vi "Checking_exe.vi"(8 "Task error in (no error)":errorcluster, 11 "Programes":string) -> (0 "Task error out":errorcluster, 3 "Game Running":bool=TRUE)   [LabVIEW 2014]
doc: "Check if an exe is running and optionally kill the process"
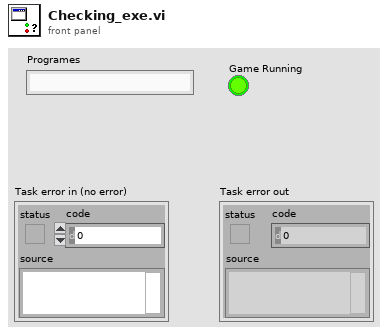
[diagram p1: front panel]
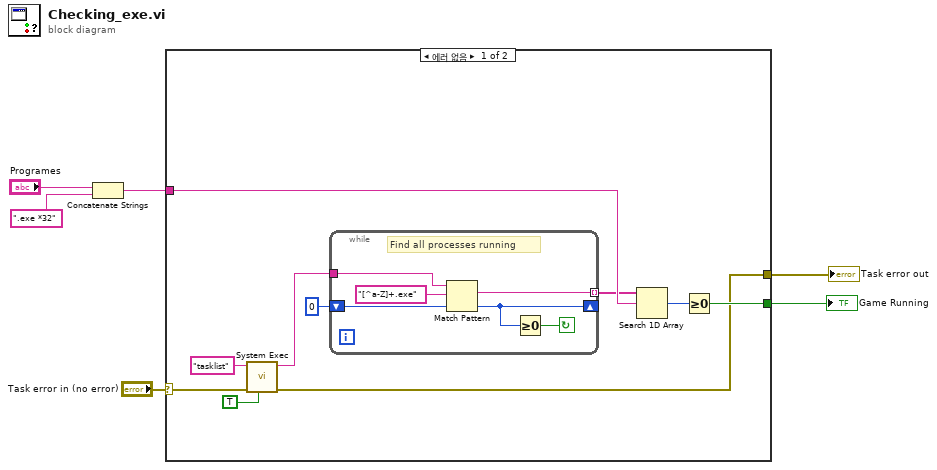
[diagram p0: block diagram]
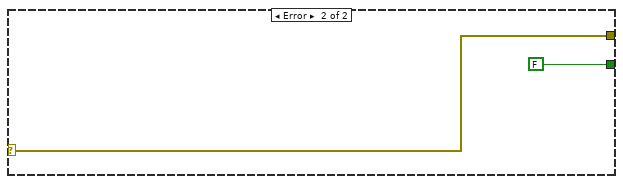
[diagram p2: hidden frame]
diagram:
  n1 = Concatenate Strings("Programes", ".exe *32") -> (w1:string)
  n2 = case shown="에러 없음" "Task error in (no error)" {
    selector: "Task error in (no error)" -> [w11 w24]
    tunnel: [w16 FALSE] -> w6
    tunnel: w1 -> [w10 _]
    tunnel: [w7 w24] -> w5
    frame No Error {
      n3 = call <vilib>:"System Exec.vi"("run minimized? (F)"=TRUE, "error in (no error)"=w11, "command line"="tasklist" ("standard input")) -> ("error out"=w7:errorcluster, "standard output"=w13:string)  [unwired: 5 in, 2 out]
      n4 = while {
        tunnel: w13 -> [w22]
        shift-right: [w18] -> _
        shift-left: 0 ("offset past match") -> [w20]
        tunnel: [w19] -> w8 mode=indexing
        stop <- w17 continue-if-true
        # "Find all processes running"
        n5 = Match Pattern(string=w22, regular expression="[^a-Z]+.exe", offset (0)=w20) -> (match substring=w19:string, offset past match=w18:i32)  [unwired: 2 out]
        n6 = Greater Or Equal To 0?(x=w18) -> (x >= 0?=w17:bool)
      }
      n7 = Search 1D Array(1D array=w8, element=w10) -> (index of element=w9:i32)  [unwired: 1 in]
      n8 = Greater Or Equal To 0?(x=w9) -> (x >= 0?=w16:bool)
    }
    frame Error {
    }
  }
  "Game Running" <- w6
  "Task error out" <- w5
